vi "JUMP.vi"(0 "speed":u16, 1 "Laser GPIB":u8=10 max=100, 2 "y-dist":i32, 3 "x-dist":i32, 4 "Disable on?":bool=TRUE, 5 "Motor GPIB":u8=6) -> ()   [LabVIEW 2010]
uses:
  <vilib>/express/express arith-compare/Formula/XNode/ExpressFormulaBlockNode.xnode
panel:
  # "JUMP<space>[Displacement]<space>[Speed]"
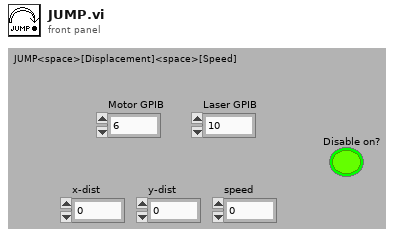
[diagram p1: front panel]
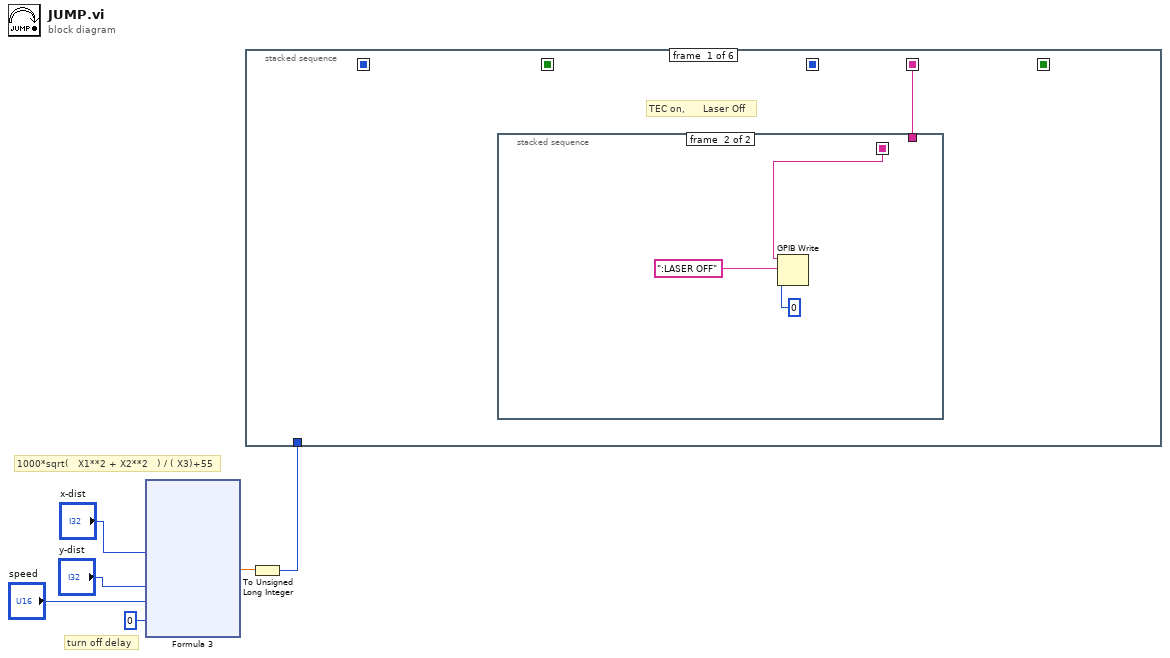
[diagram p0: block diagram]
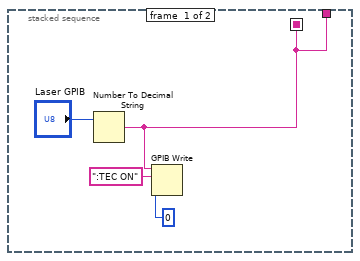
[diagram p2: hidden frame]
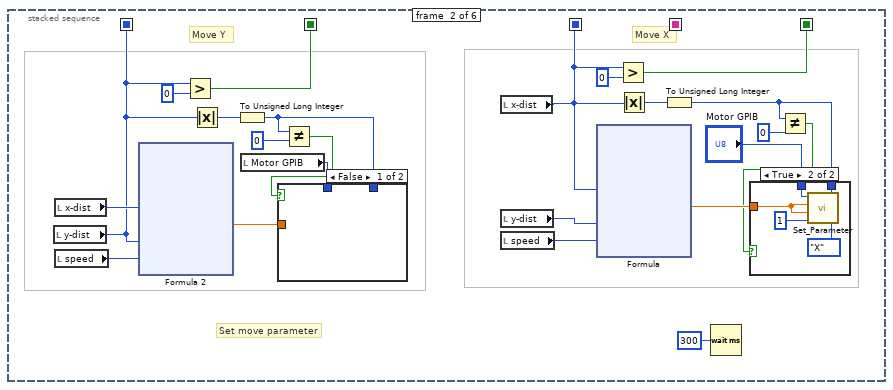
[diagram p3: hidden frame]
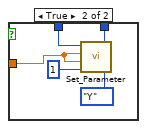
[diagram p5: hidden frame]
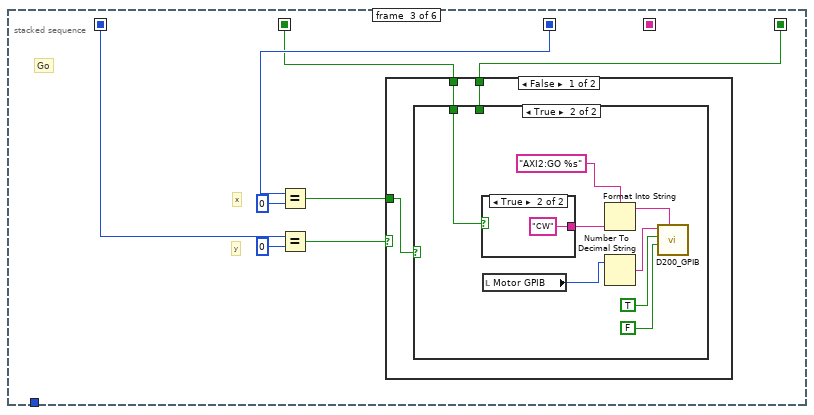
[diagram p6: hidden frame]
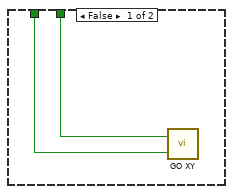
[diagram p7: hidden frame]
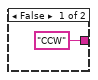
[diagram p8: hidden frame]
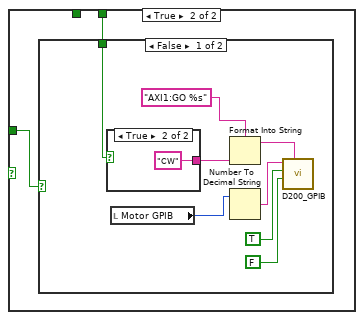
[diagram p9: hidden frame]
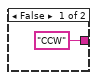
[diagram p10: hidden frame]
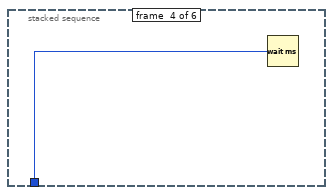
[diagram p12: hidden frame]
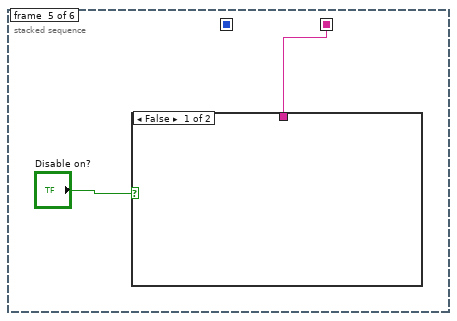
[diagram p13: hidden frame]
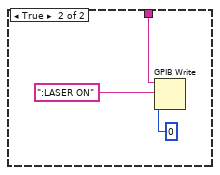
[diagram p14: hidden frame]
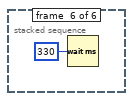
[diagram p15: hidden frame]
diagram:
  # "turn off delay"
  # "1000*sqrt(   X1**2 + X2**2   ) / ( X3)+55"
  n1 = xnode "Formula 3"("X1"="x-dist", "X2"="y-dist", "X3"="speed", "X4"=u16 0) -> ("Result"=w2:dbl)  [unwired: 1 in, 1 out]
  n2 = To Unsigned Long Integer(number=w2) -> (unsigned 32bit integer=w1:u32)
  n3 = stacked-sequence {
    seq-local: [_ w21 _ _ _ _] -> [_ _ w72 _ _ _]
    seq-local: [_ w20 _ _ _ _] -> [_ _ w73 _ _ _]
    seq-local: [_ w19 _ _ _ _] -> [_ _ w79 _ _ _]
    seq-local: [_ w18 _ _ _ _] -> [_ _ w77 _ _ _]
    seq-local: [w7 _ _ _ _ _] -> [_ _ _ _ w109 _]
    tunnel: w1 -> [_ _ _ w107 _ _]
    frame #0 {
      # "TEC on,      Laser Off"
      n4 = stacked-sequence {
        seq-local: [w8 _] -> [_ w12]
        tunnel: [w8 _] -> w7
        frame #0 {
          n5 = Number To Decimal String(number="Laser GPIB") -> (decimal integer string=w8:string)  [unwired: 1 in]
          n6 = GPIB Write(0:w8, 1:":TEC ON" ("data"), 2:i16 0 ("mode (0)")) -> ()  [unwired: 2 in, 2 out]
        }
        frame #1 {
          n7 = GPIB Write(0:w12, 1:":LASER OFF" ("data"), 2:i16 0 ("mode (0)")) -> ()  [unwired: 2 in, 2 out]
        }
      }
    }
    frame #1 {
      # "Set move parameter"
      # "Move X"
      # "Move Y"
      n8 = local read "y-dist"() -> (w19:i32)
      n9 = local read "x-dist"() -> (w34:i32)
      n10 = local read "speed"() -> (w37:u16)
      n11 = xnode "Formula 2"("X1"=w34, "X2"=w19, "X3"=w37) -> ("Result"=w29:dbl)  [unwired: 1 in, 1 out]
      n12 = Greater?(x=w19, y=0) -> (0:w21:bool)
      n13 = Absolute Value(x=w19) -> (abs(x)=w33:i32)
      n14 = To Unsigned Long Integer(number=w33) -> (unsigned 32bit integer=w27:u32)
      n15 = local read "Motor GPIB"() -> (w36:u8)
      n16 = Not Equal?(x=w27, y=u32 0) -> (x != y?=w25:bool)
      n17 = case shown="False" w25 {
        tunnel: w36 -> [_ w45]
        tunnel: w27 -> [_ w44]
        tunnel: w29 -> [_ w43]
        frame False {
        }
        frame True {
          n18 = call "Set_Parameter.vi"("Axis"=enum16{"X", "Y", "Z", "U", "V", "W"}."Y", "Distance"=w44, "Rate"=u16 1, "L Speed"=w43, "F Speed"=w43, "GPIB_Addr"=w45) -> ()
        }
      }
      n19 = local read "x-dist"() -> (w18:i32)
      n20 = local read "y-dist"() -> (w17:i32)
      n21 = local read "speed"() -> (w16:u16)
      n22 = xnode "Formula"("X1"=w18, "X2"=w17, "X3"=w16) -> ("Result"=w28:dbl)  [unwired: 1 in, 1 out]
      n23 = Greater?(x=w18, y=0) -> (0:w20:bool)
      n24 = Absolute Value(x=w18) -> (abs(x)=w30:i32)
      n25 = To Unsigned Long Integer(number=w30) -> (unsigned 32bit integer=w24:u32)
      n26 = Wait (ms)(milliseconds to wait=u32 300) -> ()  [unwired: 1 out]
      n27 = Not Equal?(x=w24, y=u32 0) -> (x != y?=w22:bool)
      n28 = case shown="True" w22 {
        tunnel: "Motor GPIB" -> [_ w42]
        tunnel: w24 -> [_ w39]
        tunnel: w28 -> [_ w38]
        frame False {
        }
        frame True {
          n29 = call "Set_Parameter.vi"("Axis"=enum16{"X", "Y", "Z", "U", "V", "W"}."X", "Distance"=w39, "Rate"=u16 1, "L Speed"=w38, "F Speed"=w38, "GPIB_Addr"=w42) -> ()
        }
      }
    }
    frame #2 {
      # "Go"
      # "x"
      # "y"
      n30 = Equal?(x=w77, y=0) -> (x = y?=w75:bool)
      n31 = Equal?(x=w79, y=0) -> (x = y?=w74:bool)
      n32 = case shown="False" w74 {
        tunnel: w75 -> [w81 w96]
        tunnel: w73 -> [w80 w95]
        tunnel: w72 -> [w82 _]
        frame False {
          n33 = case shown="True" w81 {
            tunnel: w82 -> [w84 w86]
            tunnel: w80 -> [w83 _]
            frame False {
              n34 = call "GO XY.vi"("Y-axis"=w84, "X-axis"=w83) -> ()  [unwired: 1 in]
            }
            frame True {
              n35 = case shown="True" w86 {
                tunnel: ["CCW" "CW"] -> w91
                frame False {
                }
                frame True {
                }
              }
              n36 = local read "Motor GPIB"() -> (w85:u8)
              n37 = Format Into String(format string="AXI2:GO %s", w91) -> (resulting string=w88:string)  [unwired: 2 in, 1 out]
              n38 = Number To Decimal String(number=w85) -> (decimal integer string=w87:string)  [unwired: 1 in]
              n39 = call "D200_GPIB.vi"("GPIB\nAddress"=w87, "Write"=TRUE, "Read"=FALSE, "Characters to Write"=w88) -> ()  [unwired: 1 in, 3 out]
            }
          }
        }
        frame True {
          n40 = case shown="False" w96 {
            tunnel: w95 -> [w98 _]
            frame False {
              n41 = case shown="True" w98 {
                tunnel: ["CCW" "CW"] -> w103
                frame False {
                }
                frame True {
                }
              }
              n42 = local read "Motor GPIB"() -> (w97:u8)
              n43 = Format Into String(format string="AXI1:GO %s", w103) -> (resulting string=w100:string)  [unwired: 2 in, 1 out]
              n44 = Number To Decimal String(number=w97) -> (decimal integer string=w99:string)  [unwired: 1 in]
              n45 = call "D200_GPIB.vi"("GPIB\nAddress"=w99, "Write"=TRUE, "Read"=FALSE, "Characters to Write"=w100) -> ()  [unwired: 1 in, 3 out]
            }
            frame True {
            }
          }
        }
      }
    }
    frame #3 {
      n46 = Wait (ms)(milliseconds to wait=w107) -> ()  [unwired: 1 out]
    }
    frame #4 {
      n47 = case shown="False" "Disable on?" {
        tunnel: w109 -> [_ w110]
        frame False {
        }
        frame True {
          n48 = GPIB Write(0:w110, 1:":LASER ON" ("data"), 2:i16 0 ("mode (0)")) -> ()  [unwired: 2 in, 2 out]
        }
      }
    }
    frame #5 {
      n49 = Wait (ms)(milliseconds to wait=u32 330) -> ()  [unwired: 1 out]
    }
  }
